vi "Init.vi"(8 "Project:Active Project":refnum<vi>, 9 "Application Instance":refnum<vi>, 10 "Name":string, 11 "Script Strategy in":refnum<class "Script Strategy.lvclass">) -> (3 "Script Strategy out":refnum<class "Script Strategy.lvclass">)   [LabVIEW 2021, in "_Create From Template.lvlib" / "Script Strategy.lvlib" / "Script Strategy.lvclass"]
uses:
  Script Strategy.lvclass
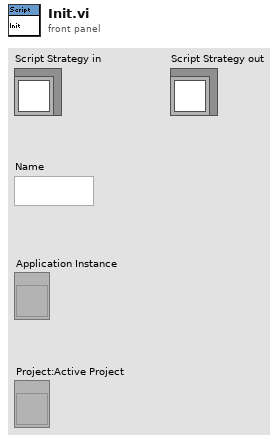
[diagram p1: front panel]
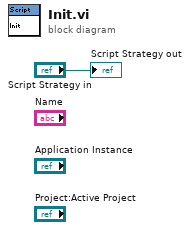
[diagram p0: block diagram]
diagram:
  "Script Strategy out" <- "Script Strategy in"
